vi "TCP Send Client.vi"() -> ()   [LabVIEW 2010]
doc: "Displays data sent via TCP from Data Server.vi. Once a TCP connection is open, the VI reads 4 bytes to determine the amount of data being sent. It then reads and charts that many bytes. If an error occurs or the stop button is pressed, it sends a \"Q\" to the Data Sender to notify it to quit.\n\n<B>Note:</B> Requires the Data Server.vi located in the same library as this VI."
uses:
  5.0-Global.vi
panel:
  in  "Address":string="10.10.10.2"
  in  "Port":u16=53483 min=1025 step=1
  # "Instructions:\n1. Open the Data Server.vi located in the same library.\n2. Follow the instructions on it's front panel.\n\nNote: This VI is built to work with the Data Server.vi."
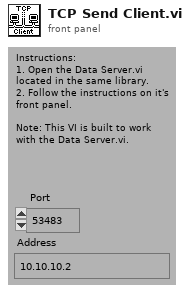
[diagram p1: front panel]
types:
  T1 = typedef "4.1-Act Control Typedef.ctl" = cluster{"4.1.0 Data":string, "Type of Data":T2, "E-Stop":bool, "Restart":bool, "Extended Joystick":bool, "Begin":bool, "Time":i32, "Shutdown":bool}
  T2 = typedef "4.1.0-Datatype Typedef.ctl" = enum16{"4.1.0-Empty Data", "4.1.1-Joystick Data", "4.1.2-Behavioral Data"}
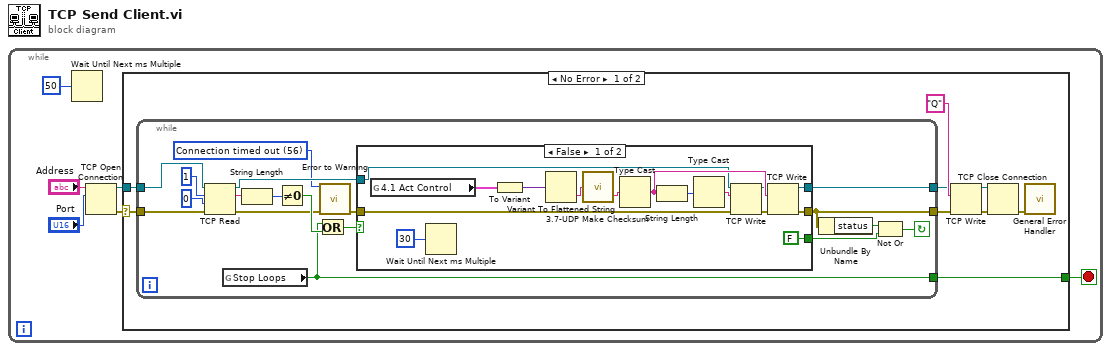
[diagram p0: block diagram]
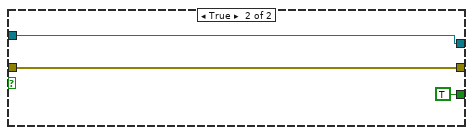
[diagram p2: hidden frame]
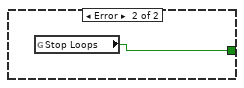
[diagram p3: hidden frame]
diagram:
  n1 = while {
    stop <- w1 stop-if-true
    n2 = Wait Until Next ms Multiple(millisecond multiple=u32 50) -> ()  [unwired: 1 out]
    n3 = TCP Open Connection(address="Address", remote port or service name="Port") -> (connection ID=w4:refnum<k5>, error out=w3:errorcluster)  [unwired: 1 in, 2 out]
    n4 = case shown="No Error" w3 {
      selector: w3 -> [w14 _]
      tunnel: w4 -> [w15 _]
      tunnel: [w7 w52] -> w1
      frame No Error {
        n5 = while {
          tunnel: [w16] -> w7
          tunnel: [w23] -> w8
          tunnel: w15 -> [w30]
          tunnel: [w18] -> w9
          tunnel: w14 -> [w17]
          stop <- w33 continue-if-true
          w21 = 56 items=["No Error", "Argument Error", "Memory Full", "Out of Zone", "End of File", "File Already Open", "Generic File IO Error", "File Not Found", "File Permission Error", "Disk Full", "Duplicate Path", "Too Many Files Open", "Not Enabled", "Resource File Not Found", "Cannot Add Resource", "Resource Not Found", "Image Not Found", "Image Memory Error", "Pen Does Not Exist", "Config Bad Type", "Config Token Not Found", "Config Parse Error", "Config Memory Error", "Bad External Code Format", "Bad External Code Offset", "External Code Not Present", "Null Window", "Destroy Window Mixup", "Null Menu", "Print Aborted", "Bad Print Record", "Print Driver Error", "Windows Error During Print", "Memory Error During Print", "Print Dialog Error", "Generic Print Error", "Invalid Device Refnum", "Device Not Found", "Device Parameter Error", "Device Unit Error", "Can't Open Device", "Device Call Aborted", "Generic Error", "Cancelled By User", "Object ID Too Low", "Object ID Too High", "Object Not In Heap", "Unknown Heap", "Bad DefProc ID", "DefProc Not In Table", "Message Out Of Range", "Null Method", "Unknown Message", "Manager Call Not Supported", "Bad address", "Connection In progress", "Connection timed out", "Connection is already in progress", "Network attribute not supported", "Network error", "Address in use", "System out of memory", "Connection aborted", "Connection refused", "Connection is not connected", "Connection is already connected", "Connection closed", "Initialize error (interapplication manager)", "Bad occurrence", "Wait on unbound occurrence handler", "Occurrence queue overflow", "Bad path", "Semaphore not signaled", "Unrecognized type (interapplication manager)"] ("1st Error to Convert")
          n6 = TCP Read(connection ID=w30, bytes to read=1, error in (no error)=w17, 9:0) -> (connection ID out=w28:refnum<k5>, data out=w29:string, error out=w20:errorcluster)  [unwired: 1 in]
          n7 = global read "5.0-Global.vi" "Stop Loops"() -> (w16:bool)
          n8 = String Length(string=w29) -> (length=w26:i32)
          n9 = Not Equal To 0?(x=w26) -> (x != 0?=w25:bool)
          n10 = Or(x=w16, y=w25) -> (x .or. y?=w24:bool)
          n11 = call <vilib>:"Error to Warning.vi"("1st Error to Convert"=w21, "error in"=w20) -> ("warning out"=w19:errorcluster)  [unwired: 13 in]
          n12 = case shown="False" w24 {
            tunnel: w19 -> [w43 w49]
            tunnel: w28 -> [w42 w50]
            tunnel: [w41 w50] -> w18
            tunnel: [w40 w49] -> w23
            tunnel: [FALSE TRUE] -> w27
            frame False {
              n13 = global read "5.0-Global.vi" "4.1 Act Control"() -> (w38:T1)
              n14 = Wait Until Next ms Multiple(millisecond multiple=u32 30) -> ()  [unwired: 1 out]
              n15 = To Variant(anything=w38) -> (Variant=w35:variant)
              n16 = Variant To Flattened String(Variant=w35) -> (data string=w37:string)  [unwired: 1 out]
              n17 = call "3.7-UDP Make Checksum.vi"("Data String In"=w37) -> ("CS String Out"=w36:string)  [unwired: 1 out]
              n18 = Type Cast(x=w36) -> (*(type *) &x=w48:string)  [unwired: 1 in]
              n19 = String Length(string=w48) -> (length=w46:i32)
              n20 = Type Cast(x=w46) -> (*(type *) &x=w47:string)  [unwired: 1 in]
              n21 = TCP Write(connection ID=w42, data in=w47, error in (no error)=w43) -> (connection ID out=w44:refnum<k5>, error out=w45:errorcluster)  [unwired: 1 in, 1 out]
              n22 = TCP Write(connection ID=w44, data in=w48, error in (no error)=w45) -> (connection ID out=w41:refnum<k5>, error out=w40:errorcluster)  [unwired: 1 in, 1 out]
            }
            frame True {
            }
          }
          n23 = Unbundle By Name(w23) -> ("status"=w22:bool)
          n24 = Not Or(1:w27, 2:w22) -> (0:w33:bool)
        }
        n25 = TCP Write(connection ID=w9, data in="Q", error in (no error)=w8) -> (connection ID out=w10:refnum<k5>, error out=w11:errorcluster)  [unwired: 2 out]
        n26 = TCP Close Connection(connection ID=w10, error in (no error)=w11) -> (error out=w13:errorcluster)  [unwired: 2 out]
        n27 = call <vilib>:"General Error Handler.vi"("error in (no error)"=w13) -> ()  [unwired: 1 in, 14 out]
      }
      frame Error {
        n28 = global read "5.0-Global.vi" "Stop Loops"() -> (w52:bool)
      }
    }
  }
